vi "Word_Quit_Graph.vi"(0 "Word.InlineShapes":refnum<k7>, 9 "Chart index":i16=-1, 11 "error in (no error)":errorcluster) -> (15 "error out":errorcluster)   [LabVIEW 2020, in "NI_ReportGenerationToolkit.lvlib"]
uses:
  <vilib>/addons/_office/NI_ReportGenerationToolkit.lvlib
panel:
  in  "Graph.Chart":refnum<k7>
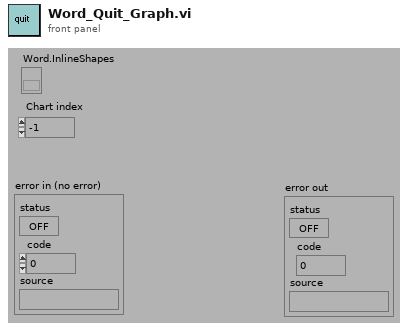
[diagram p1: front panel]
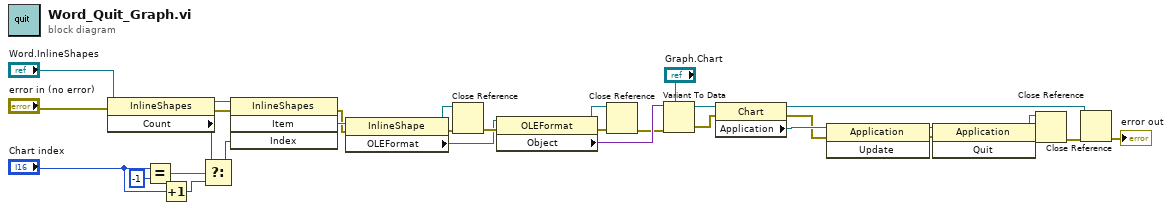
[diagram p0: block diagram]
diagram:
  n1 = property class="InlineShapes"(reference="Word.InlineShapes", error in="error in (no error)") -> (reference out=w23:refnum<k7>, error out=w31:errorcluster, "Count"=w18:i32)
  n2 = Equal?(x="Chart index", y=i16 -1) -> (x = y?=w22:bool)
  n3 = Increment(x="Chart index") -> (x+1=w20:i16)
  n4 = Select(t=w18, s=w22, f=w20) -> (s? t:f=w17:i32)
  n5 = invoke class="InlineShapes" method="Item"(reference=w23, error in=w31, "Index"=w17) -> (error out=w25:errorcluster, "Item"=w26:refnum<k7>)  [unwired: 1 in, 2 out]
  n6 = property class="InlineShape"(reference=w26, error in=w25) -> (reference out=w28:refnum<k7>, error out=w1:errorcluster, "OLEFormat"=w2:refnum<k7>)
  n7 = Close Reference(reference=w28, error in (no error)=w1) -> (error out=w27:errorcluster)
  n8 = property class="OLEFormat"(reference=w2, error in=w27) -> (reference out=w13:refnum<k7>, error out=w14:errorcluster, "Object"=w30:variant)
  n9 = Close Reference(reference=w13, error in (no error)=w14) -> (error out=w12:errorcluster)
  n10 = Variant To Data(error in=w12, type="Graph.Chart", Variant=w30) -> (data=w16:refnum<k7>, error out=w15:errorcluster)
  n11 = property class="Chart"(reference=w16, error in=w15) -> (reference out=w3:refnum<k7>, error out=w4:errorcluster, "Application"=w6:refnum<k7>)
  n12 = invoke class="Application" method="Update"(reference=w6, error in=w4) -> (reference out=w8:refnum<k7>, error out=w7:errorcluster)  [unwired: 1 in, 1 out]
  n13 = invoke class="Application" method="Quit"(reference=w8, error in=w7) -> (reference out=w10:refnum<k7>, error out=w11:errorcluster)  [unwired: 1 in, 1 out]
  n14 = Close Reference(reference=w10, error in (no error)=w11) -> (error out=w9:errorcluster)
  n15 = Close Reference(reference=w3, error in (no error)=w9) -> (error out=→"error out":errorcluster)
